vi "S2C_XML_CreateFile.vi"(8 "Error In":errorcluster) -> (0 "Error Out":errorcluster, 3 "DocRef":refnum<k20>)   [LabVIEW 2015]
uses:
  S2C_XML_Globals.vi
  <vilib>/xml/NI_XML.lvlib
  <resource>/objmgr/DOMUserDefRef.rc
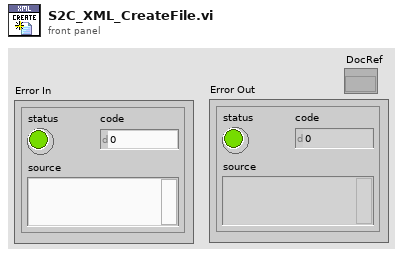
[diagram p1: front panel]
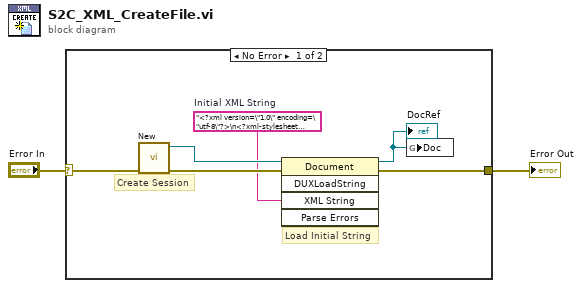
[diagram p0: block diagram]
diagram:
  n1 = case shown="No Error" "Error In" {
    selector: "Error In" -> [w5 w9]
    tunnel: [w4 w9] -> w1
    frame No Error {
      w6 = "<?xml version=\"1.0\" encoding=\"utf-8\"?>\n<?xml-stylesheet type=\"text/xsl\" href=\"IS_XML_V2.xsl\"?>\n<IntraStageXMLFile>\n<FileInfo>\n<IntraStageFileVersion>2.0</IntraStageFileVersion>\n<LastModifiedBy>Tom Armes</LastModifiedBy>\n<LastModifiedDate>3/15/2010</LastModifiedDate>\n<Comment>Covidien - KP 12/4/2013</Comment>\n</FileInfo>\n<Events>\n</Events>\n</IntraStageXMLFile>"  # Initial XML String
      # "Create Session"
      # "Load Initial String"
      n2 = call <vilib>:"New.vi"("error in (no error)"=w5) -> ("error out"=w8:errorcluster, "DOM document out"=w7:refnum<k20>)  [unwired: 7 in]
      n3 = invoke class="Document" method="DUXLoadString"(reference=w7, error in=w8, "XML String"=w6) -> (reference out=w3:refnum<k20>, error out=w4:errorcluster)  [unwired: 2 in, 3 out]
      "DocRef" <- w3
      n4 = global write "S2C_XML_Globals.vi" "Doc"(w3) -> ()
    }
    frame Error {
    }
  }
  "Error Out" <- w1
